vi "Wojtyna_B_2.vi"   [LabVIEW 2020]
uses:
  <vilib>/Platform/TimedLoop/XDataNode/timing_clust.ctl
  <vilib>/Platform/TimedLoop/XDataNode/nitl_modes.ctl
  <vilib>/Platform/TimedLoop/XDataNode/wakeup.ctl
  <vilib>/platform/TimedLoop/XDataNode/XDataNode.xnode
  <vilib>/Platform/TimedLoop/XDataNode/XDNodeRunTimeDep.lvlib
types:
  T1 = typedef "XDNodeRunTimeDep.lvlib/timing_clust.ctl" = cluster{"Expected End [f-1]":u64, "Actual End [f-1]":u64, "Finished Late? [f-1]":bool, "Expected End [i-1]":u64, "Actual End [i-1]":u64, "Finished Late? [i-1]":bool, "Expected Start [i]":u64, "Actual Start [i]":u64, "Expected Start [f]":u64, "Actual Start [f]":u64, "Source Name":string, "Structure Name":string, "Period":i64, "Deadline":i64, "Offset":i64, "Start":i64, "Priority":i32, "Timeout":i32, "Mode":T2, "Wakeup Reason":T3, "Error":errorcluster, "Source Type":string, "Secondary Source Type":string, "Global End Time":u64, "Global Start Time":u64, "Frame Duration":u64, "Iteration Duration":u64, "Assigned CPU":i32, "I/O Scan Engine Mode":u32}
  T2 = typedef "XDNodeRunTimeDep.lvlib/nitl_modes.ctl" = enum32{"No Change", "Process missed periods, maintain original phase", "Discard missed periods, maintain original phase", "Process missed periods, ignore original phase", "Discard missed periods, ignore original phase"}
  T3 = typedef "XDNodeRunTimeDep.lvlib/wakeup.ctl" = enum32{"Normal", "Aborted", "Asynchronous wakeup", "Timing source error", "Timed loop error", "Timeout"}
  T4 = typedef "Rendezvous RefNum" = refnum<k1>
  T5 = typedef "Semaphore RefNum" = refnum<k1>
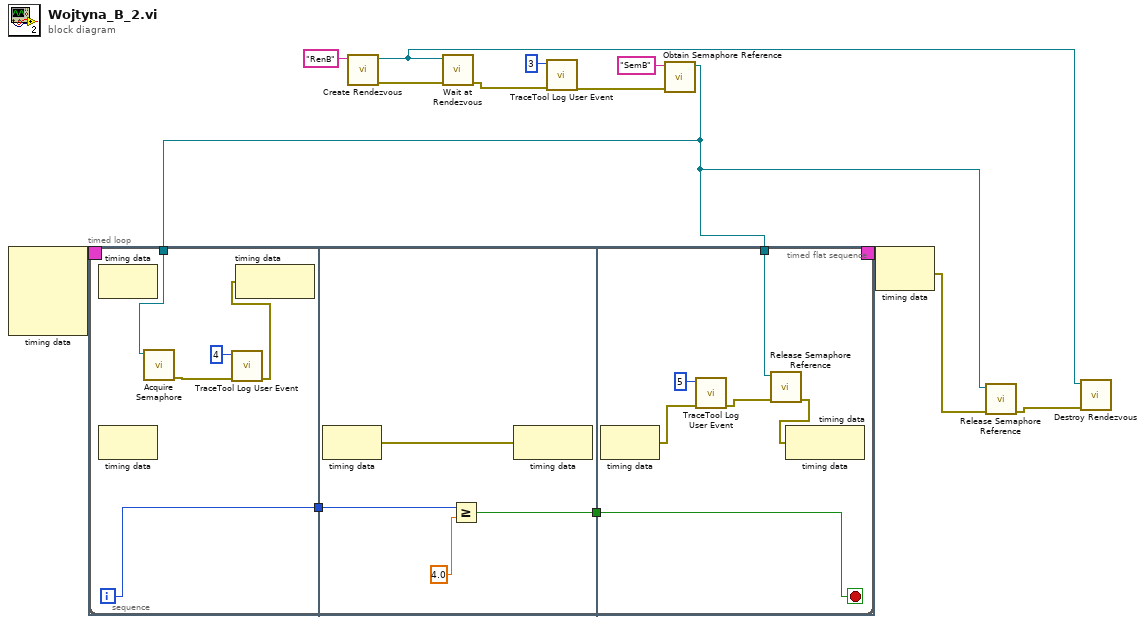
[diagram p0: block diagram]
diagram:
  n1 = node-c288() -> (w6:T1)  [unwired: 4 in]
  n2 = call <vilib>:"Create Rendezvous.vi"("name (unnamed)"="RenB") -> ("error out"=w9:errorcluster, "rendezvous"=w1:T4)  [unwired: 4 in, 1 out]
  n3 = call <vilib>:"Wait at Rendezvous.vi"("error in (no error)"=w9, "rendezvous"=w1) -> ("error out"=w10:errorcluster)  [unwired: 3 in, 2 out]
  n4 = call <vilib>:"TraceTool Log User Event.vi"("error in (no error)"=w10, "Event ID (0-255)"=u32 3) -> ("error out"=w8:errorcluster)  [unwired: 9 in]
  n5 = call <vilib>:"Obtain Semaphore Reference.vi"("error in (no error)"=w8, "name (unnamed)"="SemB") -> ("semaphore"=w2:T5)  [unwired: 3 in, 2 out]
  n6 = timed-loop {
    timing: w6 -> [_]
    timing-out: [_] -> w5
    tunnel: w2 -> [w14]
    tunnel: w2 -> [w13]
    i -> [w21]
    stop <- w42 stop-if-true
    n7 = timed-sequence {
      timing: _ -> [_]
      timing-out: _ -> [_]
      tunnel: w14 -> [w16]
      tunnel: w13 -> [w15]
      n8 = timed-flat-sequence {
        tunnel: [w21] -> w18
        tunnel: w16 -> [w19]
        tunnel: w18 -> [w30]
        tunnel: [w29] -> w17
        tunnel: w17 -> [w42]
        tunnel: w15 -> [w37]
        frame #0 {
          n9 = node-c288() -> ()  [unwired: 1 in, 1 out]
          n10 = call <vilib>:"Acquire Semaphore.vi"("semaphore"=w19) -> ("error out"=w23:errorcluster)  [unwired: 4 in, 2 out]
          n11 = call <vilib>:"TraceTool Log User Event.vi"("error in (no error)"=w23, "Event ID (0-255)"=u32 4) -> ("error out"=w20:errorcluster)  [unwired: 9 in]
          n12 = node-c288(w20) -> ()  [unwired: 1 out]
        }
        frame #1 {
          n13 = node-c288() -> (w28:errorcluster)  [unwired: 1 in]
          n14 = Greater Or Equal?(x=w30, y=4.0) -> (x >= y?=w29:bool)
          n15 = node-c288(w28) -> ()  [unwired: 1 out]
        }
        frame #2 {
          n16 = node-c288() -> (w41:errorcluster)  [unwired: 1 in]
          n17 = call <vilib>:"TraceTool Log User Event.vi"("error in (no error)"=w41, "Event ID (0-255)"=u32 5) -> ("error out"=w39:errorcluster)  [unwired: 9 in]
          n18 = call <vilib>:"Release Semaphore Reference.vi"("error in (no error)"=w39, "semaphore"=w37) -> ("error out"=w38:errorcluster)  [unwired: 8 in, 1 out]
          n19 = node-c288(w38) -> ()  [unwired: 1 out]
        }
      }
    }
    n20 = node-c288() -> ()  [unwired: 1 in, 1 out]
    n21 = node-c288() -> ()  [unwired: 1 in, 1 out]
  }
  n22 = node-c288(w5) -> (w3:errorcluster)
  n23 = call <vilib>:"Release Semaphore Reference.vi"("error in (no error)"=w3, "semaphore"=w2) -> ("error out"=w4:errorcluster)  [unwired: 8 in, 1 out]
  n24 = call <vilib>:"Destroy Rendezvous.vi"("error in (no error)"=w4, "rendezvous"=w1) -> ()  [unwired: 4 in, 2 out]
